vi "GoBang_Data2PV.vi"(8 "error in (no error)":errorcluster, 11 "Data in":variant) -> (3 "PV out":refnum<class "PV.lvclass">)   [LabVIEW 2014]
uses:
  CS++/Packages/CSPP_Core/Classes/CS++ProcessVariables/ProcessVariable/PV.lvclass
  CS++/Packages/CSPP_Core/Classes/CS++ProcessVariables/ProcessVariable/PV.lvclass/PV.ctl
  CS++/Packages/CSPP_Core/Classes/CS++ProcessVariables/ProcessVariable/Write Data.vi
  CS++/Packages/CSPP_Core/Classes/CS++ProcessVariables/ProcessVariable/Write Timestamp.vi
  CS++/Packages/CSPP_Core/Classes/CS++ProcessVariables/ProcessVariable/Write Quality.vi
  CS++/Packages/CSPP_Core/Classes/CS++ProcessVariables/ProcessVariable/Write status.vi
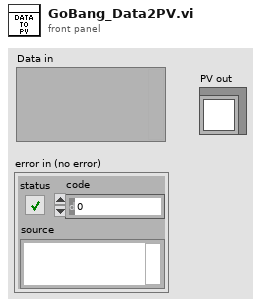
[diagram p1: front panel]
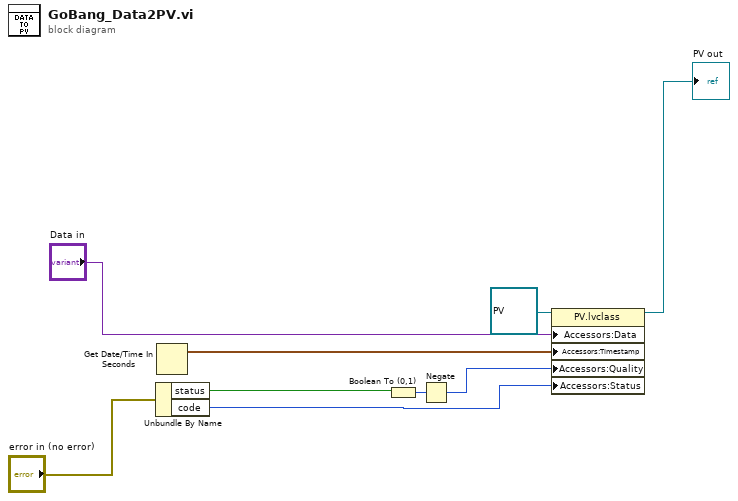
[diagram p0: block diagram]
diagram:
  n1 = Unbundle By Name("error in (no error)") -> ("status"=w3:bool, "code"=w6:i32)
  n2 = Get Date/Time In Seconds() -> (seconds since 1Jan1904=w7:timestamp)
  n3 = Boolean To (0,1)(Boolean=w3) -> (0, 1=w2:i16)
  n4 = Negate(x=w2) -> (-x=w5:i16)
  n5 = property class="PV.lvclass"(reference=refnum<class "PV.lvclass"> refnum ("CS++ProcessVariables.lvlib:PV.lvclass"), "Accessors:Data"="Data in", "Accessors:Timestamp"=w7, "Accessors:Quality"=w5, "Accessors:Status"=w6) -> (reference out=→"PV out":refnum<class "PV.lvclass">)  [unwired: 1 in, 1 out]
